vi "module create Stem.vi"(8 "error in (no error)":errorcluster, 9 "sn":u32, 10 "result":cluster{"value":i32, "error":i32}, 11 "id":u32) -> (0 "error out":errorcluster, 2 "result out":cluster{"value":i32, "error":i32}, 3 "id out":u32)   [LabVIEW 2025, in "BrainStem2_LabVIEW_Library.lvlib"]
doc: "aLIBEXPORT void __stdcall module_createStem(unsigned int* id, struct Result* result, unsigned int sn = 0);"
uses:
  BrainStem2_LabVIEW_Library.lvlib
  BrainStem2_LabVIEW.dll
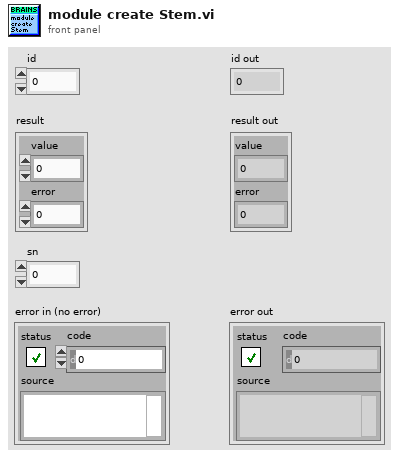
[diagram p1: front panel]
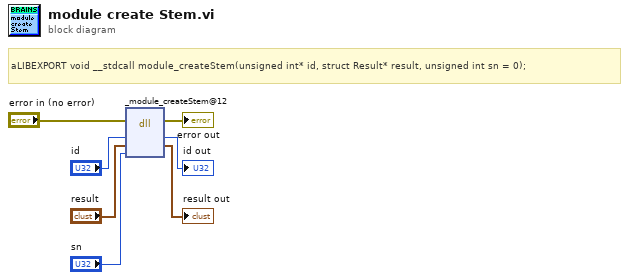
[diagram p0: block diagram]
diagram:
  # "aLIBEXPORT void __stdcall module_createStem(unsigned int* id, struct Result* result, unsigned int sn = 0);"
  n1 = dll-call lib="C:/TDS Dev/T250021 REPO/t250021-pa-module-burn-in-test/Plugins/Acroname BrainStem2 Library (KEN)/BrainStem2_LabVIEW.*" fn="_module_createStem@12"(error in="error in (no error)", "id"="id", "result"="result", "sn"="sn") -> (error out=→"error out":errorcluster, "id"=→"id out":u32, "result"=→"result out":cluster{"value":i32, "error":i32})  [unwired: 4 in, 1 out]
